vi "SegmentSequencer_Create.vi"(10 "req fifo 2":refnum<k21>, 11 "req fifo 1":refnum<k21>) -> (3 "New SegmentSequencer":refnum<class "SegmentSequencer.lvclass">)   [LabVIEW 2019, in "TX burst sequencer.lvlib" / "SegmentSequencer.lvclass"]
uses:
  SegmentSequencer.lvclass
  SegmentSequencer.lvclass/SegmentSequencer.ctl
  <vilib>/rvi/DataTransferAndStorage/Container/Common/niFpgaContainerGetUniqueNameForEmu.vi
  <vilib>/rvi/DataTransferAndStorage/Container/Common/niFpgaContainerSetEmuInfo.vi
  <vilib>/rvi/eio/common/nirviEmuReportErrorAndStop.vi
  <vilib>/rvi/LocalResourceManager/LocalResourceManager.xnode
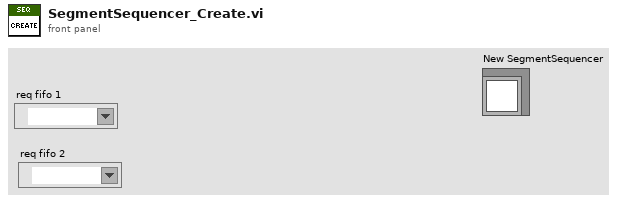
[diagram p1: front panel]
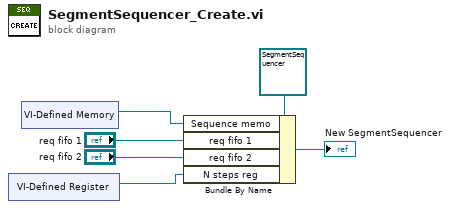
[diagram p0: block diagram]
diagram:
  n1 = xnode "VI-Defined Register"() -> ("Register Out"=w4:refnum<k21>)
  n2 = xnode "VI-Defined Memory"() -> ("Memory Out"=w2:refnum<k21>)
  n3 = Bundle By Name(cluster=refnum<class "SegmentSequencer.lvclass"> refnum ("SegmentSequencer out"), "Sequence memo"=w2, "req fifo 1"="req fifo 1", "req fifo 2"="req fifo 2", "N steps reg"=w4) -> (→"New SegmentSequencer":refnum<class "SegmentSequencer.lvclass">)
